vi "String_Type_Checker.vi"(11 "String":string) -> (1 "Number":string, 3 "Type":string)   [LabVIEW 2025, in "Table_Filtering.lvlib"]
uses:
  Table_Filtering.lvlib
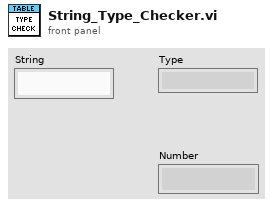
[diagram p1: front panel]
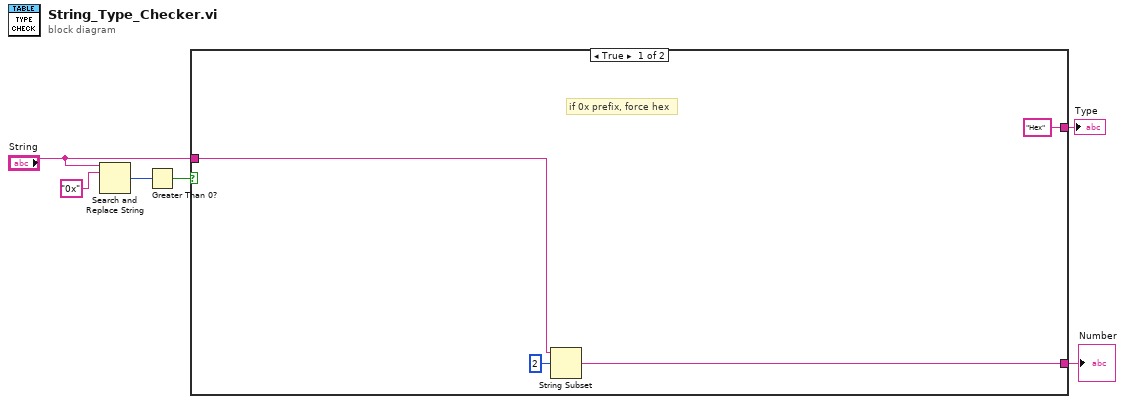
[diagram p0: block diagram]
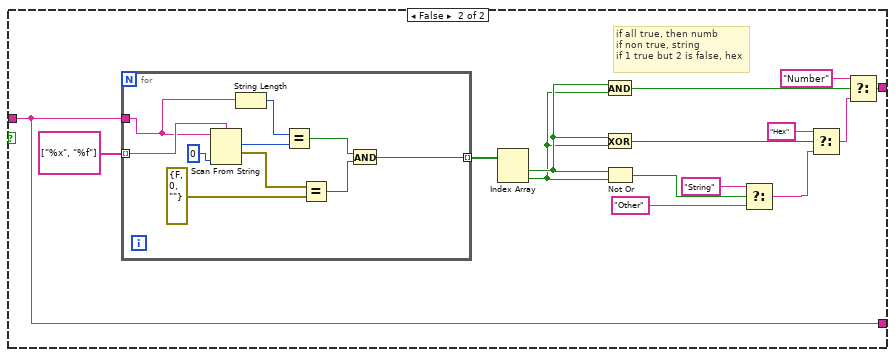
[diagram p2: hidden frame]
diagram:
  n1 = Search and Replace String(input string="String", search string="0x" ("regular expression")) -> (number of replacements=w4:i32)  [unwired: 6 in, 3 out]
  n2 = Greater Than 0?(x=w4) -> (x > 0?=w3:bool)
  n3 = case shown="True" w3 {
    tunnel: ["Hex" ("t") w15] -> w6
    tunnel: "String" -> [w9 w11]
    tunnel: [w7 w11] -> w2
    frame True {
      # "if 0x prefix, force hex"
      n4 = String Subset(string=w9, offset (0)=2) -> (substring=w7:string)  [unwired: 1 in]
    }
    frame False {
      # "if all true, then numb\nif non true, string\nif 1 true but 2 is false, hex"
      n5 = for {
        tunnel: string[] ["%x", "%f"] -> [w35] mode=indexing
        tunnel: w11 -> [w34]
        tunnel: [w27] -> w24 mode=indexing
        n6 = Scan From String(format string=w35, input string=w34, default 1=0 ("length")) -> (offset past scan=w33:u32, error out=w30:errorcluster)  [unwired: 3 in, 1 out]
        n7 = String Length(string=w34) -> (length=w32:i32)
        n8 = Equal?(x=w32, y=w33) -> (x = y?=w29:bool)
        n9 = Equal?(x=w30, y=errorcluster {"status"=FALSE, "code"=0, "source"=""} ("error constant")) -> (x = y?=w28:bool)
        n10 = And(x=w29, y=w28) -> (x .and. y?=w27:bool)
      }
      n11 = Index Array(array=w24) -> (element #1=w14:bool, element #2=w13:bool)  [unwired: 2 in]
      n12 = And(x=w14, y=w13) -> (x .and. y?=w17:bool)
      n13 = Exclusive Or(1:w13, 2:w14) -> (0:w22:bool)
      n14 = Not Or(1:w13, 2:w14) -> (0:w21:bool)
      n15 = Select(t="String", s=w21, f="Other") -> (s? t:f=w20:string)
      n16 = Select(t="Hex", s=w22, f=w20) -> (s? t:f=w18:string)
      n17 = Select(t="Number", s=w17, f=w18) -> (s? t:f=w15:string)
    }
  }
  "Type" <- w6
  "Number" <- w2
